vi "Init Stim Pattern Display.vi"(4 "Stim Pattern Values":T1[][](array[typedef]), 5 "Stim Pattern Values 2":T1[][](array[typedef])) -> (2 "Stim Pattern Display":T4)   [LabVIEW 2019]
uses:
  Controls/Muscle Group Labels.ctl
  Controls/Gait Phase Names.ctl
  Controls/Stim off-half-ful.ctl
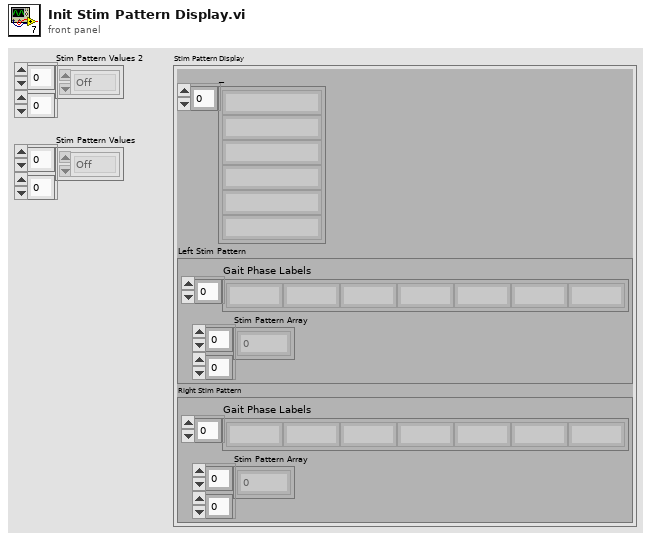
[diagram p1: front panel]
types:
  T1 = typedef "Stim off-half-ful.ctl" = enum16{"Off", "Half", "Full"}
  T2 = typedef "Muscle Group Labels.ctl" = string[]
  T3 = typedef "Gait Phase Names.ctl" = string[]
  T4 = cluster{"_":T2, "Left Stim Pattern":cluster{"Gait Phase Labels  ":T3, "Stim Pattern Array":u32[][]}, "Right Stim Pattern":cluster{"Gait Phase Labels  ":T3, "Stim Pattern Array":u32[][]}}
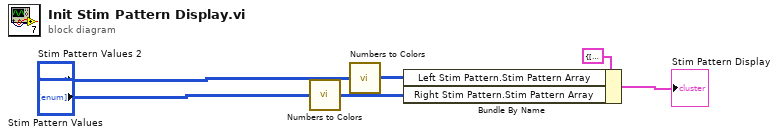
[diagram p0: block diagram]
diagram:
  n1 = call "Numbers to Colors.vi"("Left Stim Pattern Values"="Stim Pattern Values") -> ("Stim Pattern Array"=w5:u32[][])
  n2 = call "Numbers to Colors.vi"("Left Stim Pattern Values"="Stim Pattern Values 2") -> ("Stim Pattern Array"=w3:u32[][])
  n3 = Bundle By Name(cluster=T4 {"_"=["Muscle Groups", "Gluteals", "Hamstrings", "Quadriceps", "Tibialis Anterior", "Triceps Surae"], "Left Stim Pattern"={"Gait Phase Labels  "=["LR", "MSt", "TSt", "PSw", "ISw", "MSw", "TSw"], "Stim Pattern Array"=[]}, "Right Stim Pattern"={"Gait Phase Labels  "=["LR", "MSt", "TSt", "PSw", "ISw", "MSw", "TSw"], "Stim Pattern Array"=[]}} ("Stim Pattern Display"), "Left Stim Pattern.Stim Pattern Array"=w3, "Right Stim Pattern.Stim Pattern Array"=w5) -> (→"Stim Pattern Display":T4)
